vi "ParaSet.vi"(8 "error in (no error)":errorcluster, 11 "Programing Logic in":refnum<class "Programing Logic.lvclass">) -> (0 "error out":errorcluster, 3 "Programing Logic out":refnum<class "Programing Logic.lvclass">)   [LabVIEW 2014, in "Programing Logic.lvclass"]
uses:
  Programing Logic.lvclass
  Programing Logic.lvclass/Programing Logic.ctl
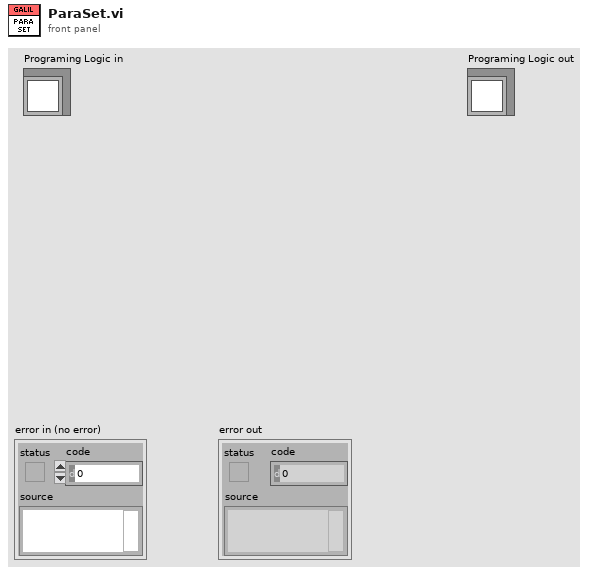
[diagram p1: front panel]
types:
  T1 = cluster{"Winding Speed":string, "Winding Length":string, "Winding Unit":string}
  T2 = cluster{"Kink Cycles":string, "Binding Length":string, "Binding Unit":string}
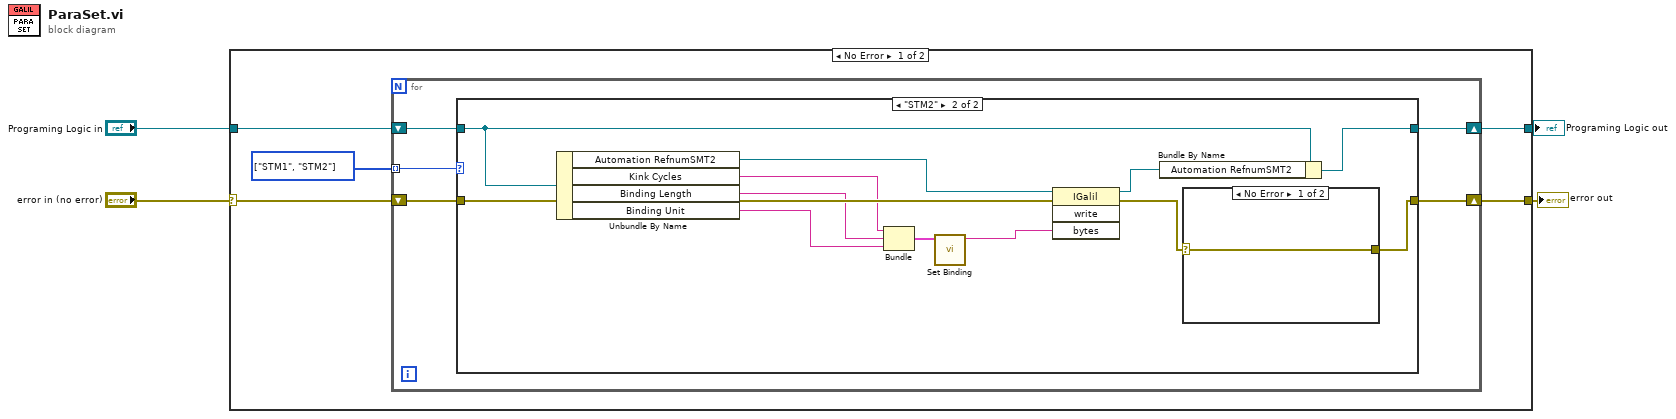
[diagram p0: block diagram]
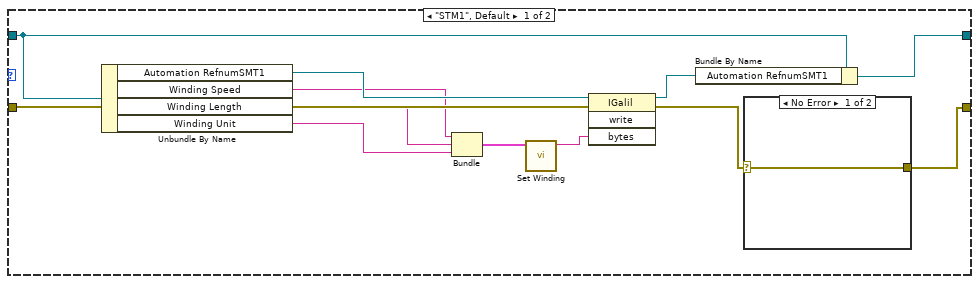
[diagram p2: hidden frame]
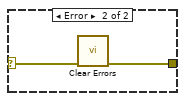
[diagram p3: hidden frame]
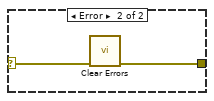
[diagram p4: hidden frame]
diagram:
  n1 = case shown="No Error" "error in (no error)" {
    selector: "error in (no error)" -> [w8 w46]
    tunnel: [w6 w46] -> w3
    tunnel: [w7 w45] -> w1
    tunnel: "Programing Logic in" -> [w9 w45]
    frame No Error {
      w5 = enum16{"STM1", "STM2", ""}[] [enum."STM1", enum."STM2"] items=["STM1", "STM2", ""]
      n2 = for {
        shift-right: [w12] -> w7
        shift-left: w9 -> [w14]
        shift-right: [w11] -> w6
        shift-left: w8 -> [w13]
        tunnel: w5 -> [w10] mode=indexing
        n3 = case shown="\"STM2\"" w10 {
          tunnel: w14 -> [w23 w40]
          tunnel: w13 -> [w24 w38]
          tunnel: [w22 w37] -> w12
          tunnel: [w15 w30] -> w11
          frame "STM1", Default {
            n4 = Unbundle By Name(w23) -> ("Automation RefnumSMT1"=w25:refnum<k7>, "Winding Speed"=w19:string, "Winding Length"=w18:string, "Winding Unit"=w17:string)
            n5 = Bundle("Winding Speed"=w19, "Winding Length"=w18, "Winding Unit"=w17) -> (w21:T1)  [unwired: 1 in]
            n6 = call "Set Winding.vi"("Recipes.Winding"=w21) -> ("concatenated string"=w20:string)  [unwired: 10 in]
            n7 = invoke class="IGalil" method="write"(reference=w25, error in=w24, "bytes"=w20) -> (reference out=w26:refnum<k7>, error out=w16:errorcluster)  [unwired: 1 in, 2 out]
            n8 = Bundle By Name(cluster=w23, "Automation RefnumSMT1"=w26) -> (w22:refnum<class "Programing Logic.lvclass">)
            n9 = case shown="No Error" w16 {
              selector: w16 -> [w27 w29]
              tunnel: [w27 w28] -> w15
              frame No Error {
              }
              frame Error {
                n10 = call <vilib>:"Clear Errors.vi"("error in (no error)"=w29) -> ("error out"=w28:errorcluster)  [unwired: 5 in, 1 out]
              }
            }
          }
          frame "STM2" {
            n11 = Unbundle By Name(w40) -> ("Automation RefnumSMT2"=w41:refnum<k7>, "Kink Cycles"=w35:string, "Binding Length"=w34:string, "Binding Unit"=w33:string)
            n12 = Bundle("Kink Cycles"=w35, "Binding Length"=w34, "Binding Unit"=w33) -> (w32:T2)  [unwired: 1 in]
            n13 = call "Set Binding.vi"("Recipes.Binding"=w32) -> ("concatenated string"=w36:string)  [unwired: 10 in]
            n14 = invoke class="IGalil" method="write"(reference=w41, error in=w38, "bytes"=w36) -> (reference out=w39:refnum<k7>, error out=w31:errorcluster)  [unwired: 1 in, 2 out]
            n15 = Bundle By Name(cluster=w40, "Automation RefnumSMT2"=w39) -> (w37:refnum<class "Programing Logic.lvclass">)
            n16 = case shown="No Error" w31 {
              selector: w31 -> [w42 w43]
              tunnel: [w42 w44] -> w30
              frame No Error {
              }
              frame Error {
                n17 = call <vilib>:"Clear Errors.vi"("error in (no error)"=w43) -> ("error out"=w44:errorcluster)  [unwired: 5 in, 1 out]
              }
            }
          }
        }
      }
    }
    frame Error {
    }
  }
  "error out" <- w3
  "Programing Logic out" <- w1
